vi "Read Write Data.vi"(7 "Enum":T2, 8 "error in (no error)":errorcluster, 9 "Sign In Detail":string[](array[string]), 10 "User Information In":T1(array[cluster]), 11 "file path":path) -> (0 "error out":errorcluster, 1 "Boolean":bool, 2 "User Information Out":T1(array[cluster]), 3 "Numeric":i32)   [LabVIEW 2013]
uses:
  Controls/Log Data Staus.ctl
  <vilib>/Utility/file.llb/Read From Spreadsheet File (string).vi
  <vilib>/Utility/file.llb/Write To Spreadsheet File (string).vi
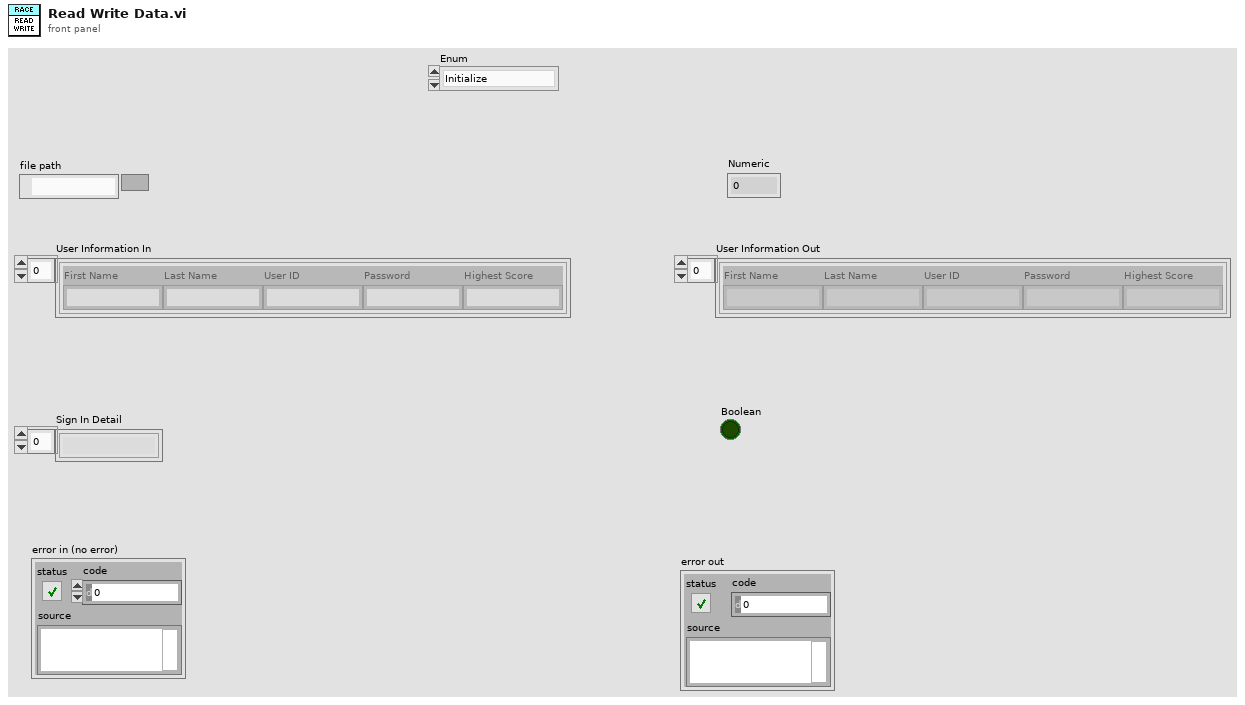
[diagram p1: front panel]
types:
  T1 = cluster{"First Name":string, "Last Name":string, "User ID":string, "Password":string, "Highest Score":string}[]
  T2 = typedef "Log Data Staus.ctl" = enum16{"Initialize", "Read", "User ID Check", "Write", "Stop"}
  T3 = cluster{"First Name":string, "Last Name":string, "User ID":string, "Password":string, "Highest Score":string}
  T4 = cluster{"First Name":string, "Last Name":string, "Account No.":string, "Password":string, "Highest Score":string}[]
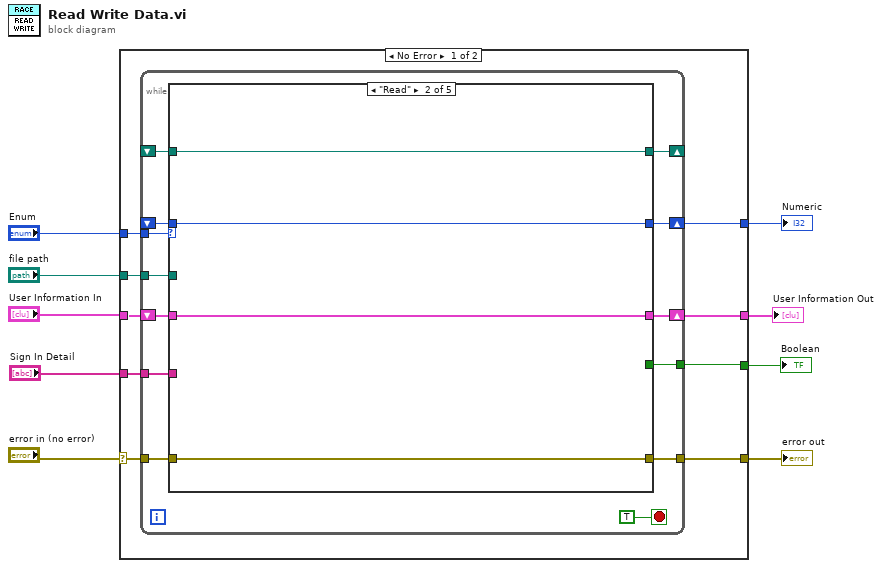
[diagram p0: block diagram]
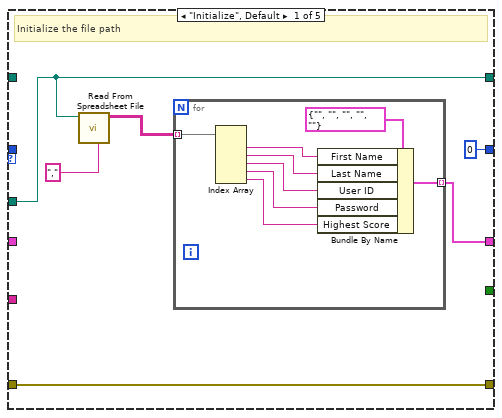
[diagram p2: hidden frame]
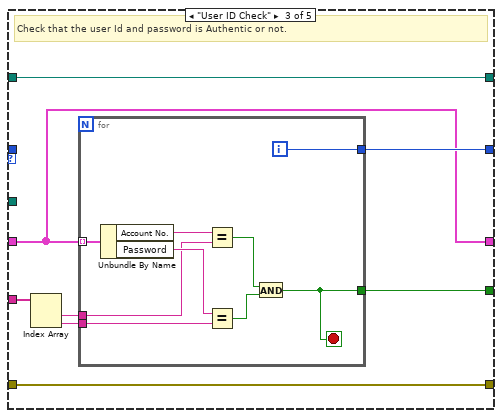
[diagram p3: hidden frame]
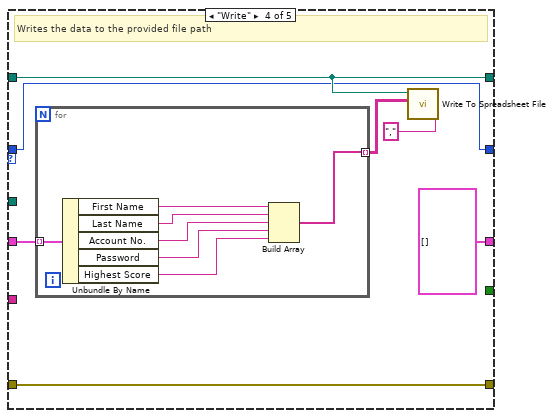
[diagram p4: hidden frame]
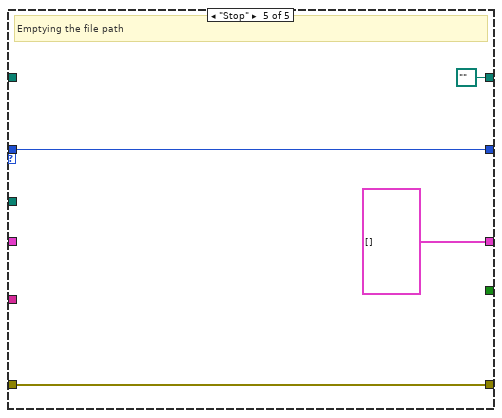
[diagram p5: hidden frame]
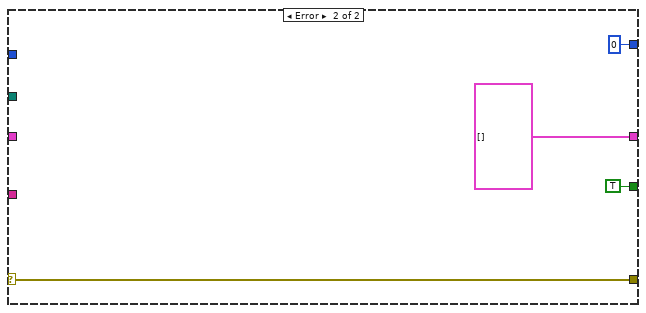
[diagram p6: hidden frame]
diagram:
  n1 = case shown="No Error" "error in (no error)" {
    selector: "error in (no error)" -> [w15 w88]
    tunnel: "Enum" -> [w18 _]
    tunnel: "file path" -> [w17 _]
    tunnel: [w13 T4 [] ("User Information In")] -> w4
    tunnel: "User Information In" -> [w16 _]
    tunnel: [w14 w88] -> w9
    tunnel: [w12 TRUE] -> w3
    tunnel: [w11 0] -> w2
    tunnel: "Sign In Detail" -> [w10 _]
    frame No Error {
      n2 = while {
        tunnel: w18 -> [w30]
        tunnel: w17 -> [w29]
        shift-right: [w28] -> _
        shift-left: _ -> [w27]
        tunnel: w15 -> [w25]
        tunnel: [w24] -> w14
        shift-right: [w23] -> w13
        shift-left: w16 -> [w26]
        tunnel: [w22] -> w12
        tunnel: w10 -> [w20]
        shift-right: [w21] -> w11
        shift-left: _ -> [w19]
        stop <- TRUE stop-if-true
        n3 = case shown="\"Read\"" w30 {
          tunnel: w29 -> [w33 _ _ _ _]
          tunnel: [w33 w48 w56 w73 path "" ("file path")] -> w28
          tunnel: w27 -> [_ w48 w56 w73 _]
          tunnel: [w34 w47 w50 T4 [] ("User Information In") T4 [] ("User Information In")] -> w23
          tunnel: w26 -> [_ w47 w50 w70 _]
          tunnel: w25 -> [w37 w49 w57 w71 w84]
          tunnel: [w37 w49 w57 w71 w84] -> w24
          tunnel: [_ _ w55 _ _] -> w22
          tunnel: [0 w46 w54 w69 w81] -> w21
          tunnel: w20 -> [_ _ w53 _ _]
          tunnel: w19 -> [_ w46 _ w69 w81]
          frame "Initialize", Default {
            # "Initialize the file path"
            n4 = call-poly <vilib>:"Read From Spreadsheet File.vi"("delimiter (\\t)"="," ("delimiter (\\t)"), "file path (dialog if empty)"=w33) -> ("all rows"=w35:string[][])  [unwired: 5 in, 4 out]
            n5 = for {
              tunnel: [w41] -> w34 mode=indexing
              tunnel: w35 -> [w40] mode=indexing
              n6 = Index Array(array=w40) -> (element #1=w44:string, element #2=w43:string, element #3=w42:string, element #4=w39:string, element #5=w38:string)  [unwired: 5 in]
              n7 = Bundle By Name(cluster=T3 {"First Name"="", "Last Name"="", "User ID"="", "Password"="", "Highest Score"=""}, "First Name"=w44, "Last Name"=w43, "User ID"=w42, "Password"=w39, "Highest Score"=w38) -> (w41:T3)
            }
          }
          frame "Read" {
          }
          frame "User ID Check" {
            # "Check that the user Id and password is Authentic or not."
            n8 = Index Array(array=w53) -> (element #1=w52:string, element #2=w51:string)  [unwired: 2 in]
            n9 = for {
              tunnel: w50 -> [w66] mode=indexing
              tunnel: [w61] -> w55
              tunnel: [w60] -> w54
              tunnel: w52 -> [w59]
              tunnel: w51 -> [w58]
              i -> [w60]
              stop <- w61 stop-if-true
              n10 = Unbundle By Name(w66) -> ("Account No."=w65:string, "Password"=w64:string)
              n11 = Equal?(x=w65, y=w59) -> (x = y?=w63:bool)
              n12 = Equal?(x=w64, y=w58) -> (x = y?=w62:bool)
              n13 = And(x=w63, y=w62) -> (x .and. y?=w61:bool)
            }
          }
          frame "Write" {
            # "Writes the data to the provided file path"
            n14 = for {
              tunnel: w70 -> [w80] mode=indexing
              tunnel: [w76] -> w72 mode=indexing
              n15 = Unbundle By Name(w80) -> ("First Name"=w79:string, "Last Name"=w78:string, "Account No."=w77:string, "Password"=w75:string, "Highest Score"=w74:string)
              n16 = Build Array(w79, w78, w77, w75, w74) -> (w76:string[])
            }
            n17 = call-poly <vilib>:"Write To Spreadsheet File.vi"("delimiter (\\t)"="," ("delimiter (\\t)"), "2D data"=w72, "file path (dialog if empty)"=w73) -> ()  [unwired: 5 in, 1 out]
          }
          frame "Stop" {
            # "Emptying the file path"
          }
        }
      }
    }
    frame Error {
    }
  }
  "error out" <- w9
  "User Information Out" <- w4
  "Boolean" <- w3
  "Numeric" <- w2
